vi "Multi Dut Cmd_Header Setting.vi"(8 "error in (no error)":errorcluster, 9 "Test Seq":i32(ring) items=["C1_C2_C3", "C2_C1_C3", "C3_C2_C1"], 11 "WS1050/51":bool=TRUE) -> (0 "error out":errorcluster, 1 "Cmd 3":string[](array[string]), 2 "Name 3":string[](array[string]), 3 "Name Header":string[](array[string]), 4 "Cmd 2":string[](array[string]), 5 "Name 2":string[](array[string]), 6 "Cmd 1":string[](array[string]), 7 "Name 1":string[](array[string]))   [LabVIEW 2012]
panel:
  in  "Cmd 51":string[](array[string])=["00", "01", "00", "02", "00", "04", "00", "08", "04", "0C", "08", "10", "0C", "14", "10", "18", "14", "1C", "18", "20", "1C", "24", "20", "28", "24", "2C", "28", "2F", "00"]
  in  "Name 51":string[](array[string])=["Min", "F1", "F1_OFF", "F2", "F2_OFF", "S1", "S1_OFF", "S2", "S2_OFF", "S3", "S3_OFF", "S4", "S4_OFF", "S5", "S5_OFF", "S6", "S6_OFF", "S7", "S7_OFF", "S8", "S8_OFF", "S9", "S9_OFF", "S10", "S10_OFF", "S11", "S11_OFF", "S11_F12", "Min2"]
  in  "Cmd 50":string[](array[string])=["00", "01", "00", "02", "00", "04", "00", "08", "04", "0C", "08", "10", "0C", "14", "10", "18", "14", "1C", "18", "20", "1C", "24", "20", "28", "24", "2C", "28", "30", "2C", "34", "30", "38", "34", "3B", "00"]
  in  "Name 50":string[](array[string])=["Min", "F1", "F1_OFF", "F2", "F2_OFF", "S1", "S1_OFF", "S2", "S2_OFF", "S3", "S3_OFF", "S4", "S4_OFF", "S5", "S5_OFF", "S6", "S6_OFF", "S7", "S7_OFF", "S8", "S8_OFF", "S9", "S9_OFF", "S10", "S10_OFF", "S11", "S11_OFF", "S12", "S12_OFF", "S13", "S13_OFF", "S14", "S14_OFF", "S14F12", "Min2"]
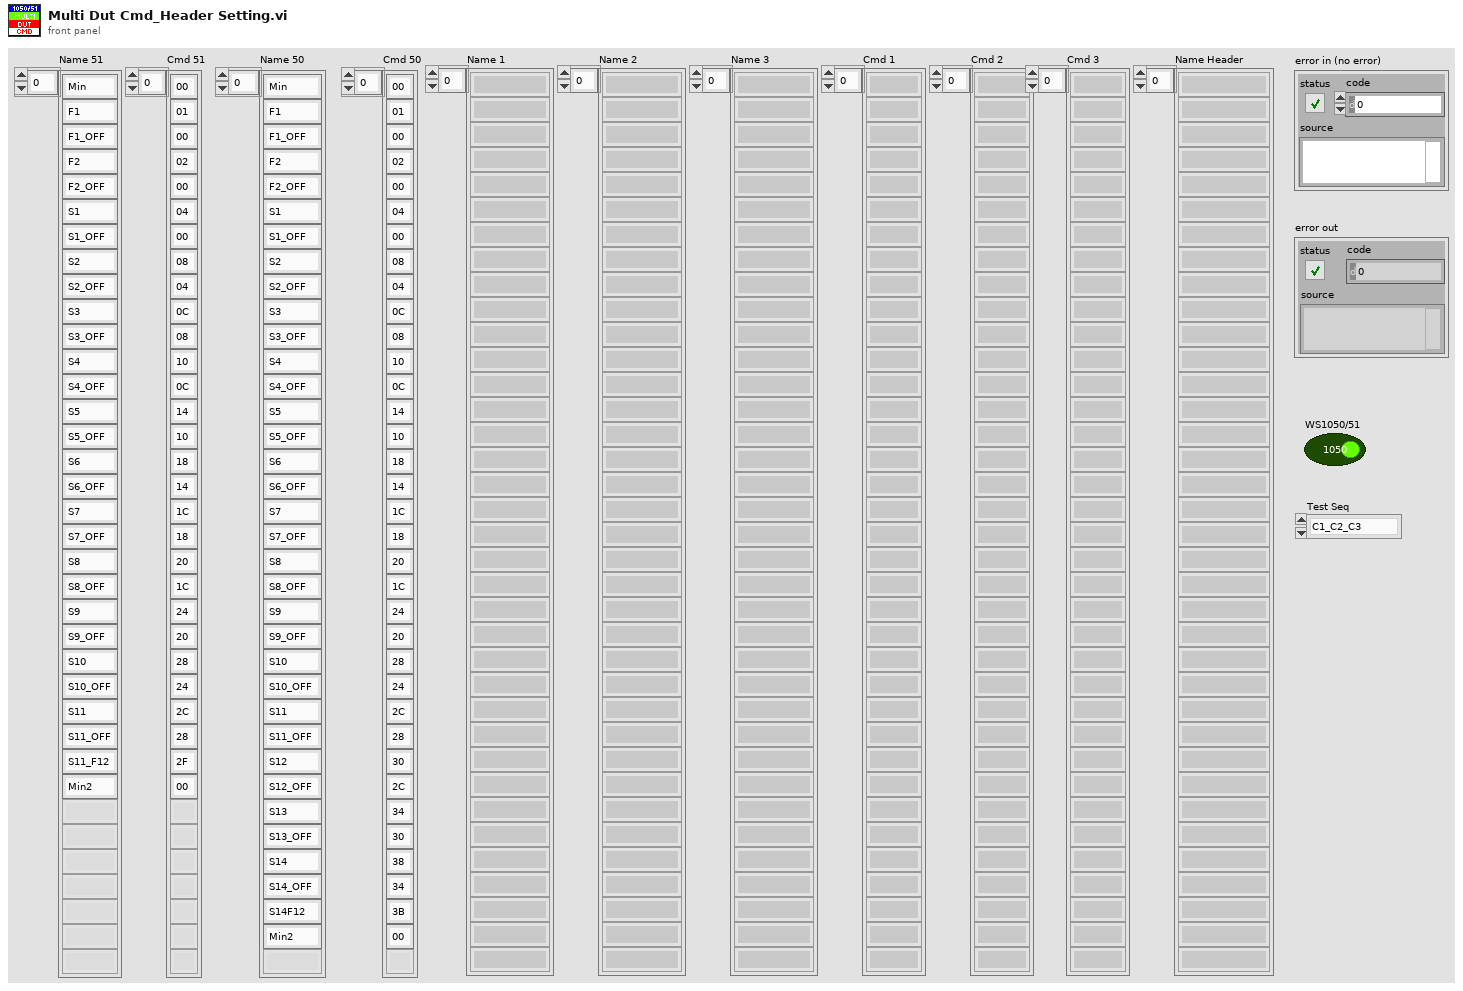
[diagram p1: front panel]
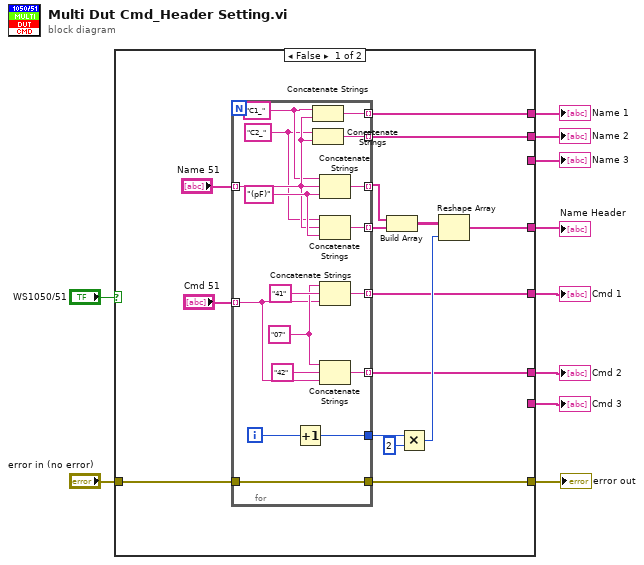
[diagram p0: block diagram]
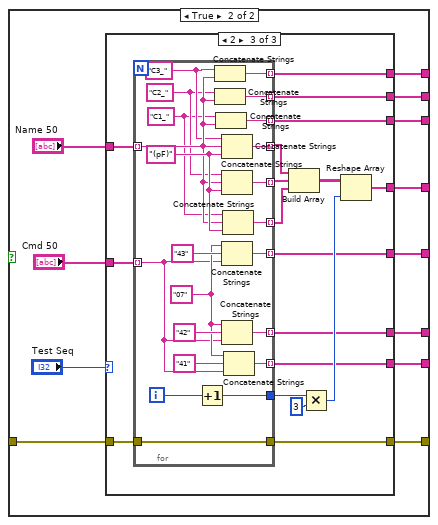
[diagram p2: hidden frame]
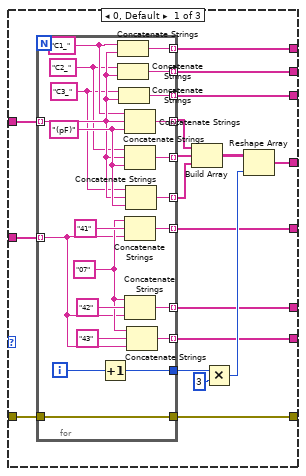
[diagram p3: hidden frame]
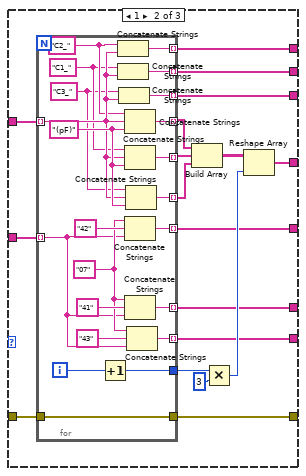
[diagram p4: hidden frame]
diagram:
  n1 = case shown="False" "WS1050/51" {
    tunnel: "error in (no error)" -> [w14 w52]
    tunnel: [w13 w51] -> w9
    tunnel: [w17 w50] -> w7
    tunnel: [w19 w49] -> w6
    tunnel: [w18 w48] -> w5
    tunnel: [_ w47] -> w4
    tunnel: [w12 w46] -> w3
    tunnel: [w11 w45] -> w2
    tunnel: [_ w44] -> w1
    frame False {
      n2 = for {
        tunnel: "Name 51" -> [w29] mode=indexing
        tunnel: [w42] -> w20 mode=indexing
        tunnel: [w41] -> w21 mode=indexing
        tunnel: "Cmd 51" -> [w35] mode=indexing
        tunnel: [w39] -> w12 mode=indexing
        tunnel: [w37] -> w11 mode=indexing
        tunnel: [w31] -> w19 mode=indexing
        tunnel: [w33] -> w24
        tunnel: [w30] -> w18 mode=indexing
        tunnel: w14 -> [w26]
        tunnel: [w26] -> w13
        i -> [w32]
        w27 = "C2_" ("string")
        w34 = "(pF)" ("string")
        w28 = "C1_" ("string")
        w36 = "07" ("string")
        n3 = Increment(x=w32) -> (x+1=w33:i32)
        n4 = Concatenate Strings(w28, w29) -> (w31:string)
        n5 = Concatenate Strings(w27, w29) -> (w30:string)
        n6 = Concatenate Strings(w28, w29, w34) -> (w42:string)
        n7 = Concatenate Strings(w27, w29, w34) -> (w41:string)
        n8 = Concatenate Strings(w36, "41" ("string"), w35) -> (w39:string)
        n9 = Concatenate Strings(w36, "42" ("string"), w35) -> (w37:string)
      }
      n10 = Build Array(w20, w21) -> (w22:string[][])
      n11 = Multiply(x=w24, y=2) -> (x*y=w23:i32)
      n12 = Reshape Array(w22, w23) -> (w17:string[])
    }
    frame True {
      n13 = case shown="2" "Test Seq" {
        tunnel: "Name 50" -> [w72 w112 w152]
        tunnel: "Cmd 50" -> [w71 w111 w151]
        tunnel: w52 -> [w63 w103 w143]
        tunnel: [w62 w102 w142] -> w51
        tunnel: [w61 w101 w141] -> w50
        tunnel: [w60 w100 w140] -> w49
        tunnel: [w59 w99 w139] -> w48
        tunnel: [w58 w98 w138] -> w47
        tunnel: [w57 w97 w137] -> w46
        tunnel: [w56 w96 w136] -> w45
        tunnel: [w55 w95 w135] -> w44
        frame 0, Default {
          n14 = for {
            tunnel: w72 -> [w78] mode=indexing
            tunnel: [w94] -> w70 mode=indexing
            tunnel: [w93] -> w69 mode=indexing
            tunnel: [w92] -> w68 mode=indexing
            tunnel: w71 -> [w85] mode=indexing
            tunnel: [w90] -> w57 mode=indexing
            tunnel: [w88] -> w56 mode=indexing
            tunnel: [w84] -> w55 mode=indexing
            tunnel: [w80] -> w60 mode=indexing
            tunnel: [w82] -> w65
            tunnel: [w79] -> w59 mode=indexing
            tunnel: [w77] -> w58 mode=indexing
            tunnel: w63 -> [w73]
            tunnel: [w73] -> w62
            i -> [w81]
            w74 = "C3_" ("string")
            w75 = "C2_" ("string")
            w83 = "(pF)" ("string")
            w76 = "C1_" ("string")
            w87 = "07" ("string")
            n15 = Increment(x=w81) -> (x+1=w82:i32)
            n16 = Concatenate Strings(w76, w78) -> (w80:string)
            n17 = Concatenate Strings(w75, w78) -> (w79:string)
            n18 = Concatenate Strings(w74, w78) -> (w77:string)
            n19 = Concatenate Strings(w76, w78, w83) -> (w94:string)
            n20 = Concatenate Strings(w75, w78, w83) -> (w93:string)
            n21 = Concatenate Strings(w87, "41" ("string"), w85) -> (w90:string)
            n22 = Concatenate Strings(w87, "42" ("string"), w85) -> (w88:string)
            n23 = Concatenate Strings(w74, w78, w83) -> (w92:string)
            n24 = Concatenate Strings(w87, "43" ("string"), w85) -> (w84:string)
          }
          n25 = Build Array(w70, w69, w68) -> (w67:string[][])
          n26 = Multiply(x=w65, y=3) -> (x*y=w66:i32)
          n27 = Reshape Array(w67, w66) -> (w61:string[])
        }
        frame 1 {
          n28 = for {
            tunnel: w112 -> [w118] mode=indexing
            tunnel: [w134] -> w110 mode=indexing
            tunnel: [w133] -> w109 mode=indexing
            tunnel: [w132] -> w108 mode=indexing
            tunnel: w111 -> [w125] mode=indexing
            tunnel: [w130] -> w97 mode=indexing
            tunnel: [w128] -> w96 mode=indexing
            tunnel: [w124] -> w95 mode=indexing
            tunnel: [w120] -> w100 mode=indexing
            tunnel: [w122] -> w105
            tunnel: [w119] -> w99 mode=indexing
            tunnel: [w117] -> w98 mode=indexing
            tunnel: w103 -> [w113]
            tunnel: [w113] -> w102
            i -> [w121]
            w114 = "C3_" ("string")
            w115 = "C1_" ("string")
            w123 = "(pF)" ("string")
            w116 = "C2_" ("string")
            w127 = "07" ("string")
            n29 = Increment(x=w121) -> (x+1=w122:i32)
            n30 = Concatenate Strings(w116, w118) -> (w120:string)
            n31 = Concatenate Strings(w115, w118) -> (w119:string)
            n32 = Concatenate Strings(w114, w118) -> (w117:string)
            n33 = Concatenate Strings(w116, w118, w123) -> (w134:string)
            n34 = Concatenate Strings(w115, w118, w123) -> (w133:string)
            n35 = Concatenate Strings(w127, "42" ("string"), w125) -> (w130:string)
            n36 = Concatenate Strings(w127, "41" ("string"), w125) -> (w128:string)
            n37 = Concatenate Strings(w114, w118, w123) -> (w132:string)
            n38 = Concatenate Strings(w127, "43" ("string"), w125) -> (w124:string)
          }
          n39 = Build Array(w110, w109, w108) -> (w107:string[][])
          n40 = Multiply(x=w105, y=3) -> (x*y=w106:i32)
          n41 = Reshape Array(w107, w106) -> (w101:string[])
        }
        frame 2 {
          n42 = for {
            tunnel: w152 -> [w158] mode=indexing
            tunnel: [w174] -> w150 mode=indexing
            tunnel: [w173] -> w149 mode=indexing
            tunnel: [w172] -> w148 mode=indexing
            tunnel: w151 -> [w165] mode=indexing
            tunnel: [w170] -> w137 mode=indexing
            tunnel: [w168] -> w136 mode=indexing
            tunnel: [w164] -> w135 mode=indexing
            tunnel: [w160] -> w140 mode=indexing
            tunnel: [w162] -> w145
            tunnel: [w159] -> w139 mode=indexing
            tunnel: [w157] -> w138 mode=indexing
            tunnel: w143 -> [w153]
            tunnel: [w153] -> w142
            i -> [w161]
            w154 = "C1_" ("string")
            w155 = "C2_" ("string")
            w163 = "(pF)" ("string")
            w156 = "C3_" ("string")
            w167 = "07" ("string")
            n43 = Increment(x=w161) -> (x+1=w162:i32)
            n44 = Concatenate Strings(w156, w158) -> (w160:string)
            n45 = Concatenate Strings(w155, w158) -> (w159:string)
            n46 = Concatenate Strings(w154, w158) -> (w157:string)
            n47 = Concatenate Strings(w156, w158, w163) -> (w174:string)
            n48 = Concatenate Strings(w155, w158, w163) -> (w173:string)
            n49 = Concatenate Strings(w167, "43" ("string"), w165) -> (w170:string)
            n50 = Concatenate Strings(w167, "42" ("string"), w165) -> (w168:string)
            n51 = Concatenate Strings(w154, w158, w163) -> (w172:string)
            n52 = Concatenate Strings(w167, "41" ("string"), w165) -> (w164:string)
          }
          n53 = Build Array(w150, w149, w148) -> (w147:string[][])
          n54 = Multiply(x=w145, y=3) -> (x*y=w146:i32)
          n55 = Reshape Array(w147, w146) -> (w141:string[])
        }
      }
    }
  }
  "error out" <- w9
  "Name Header" <- w7
  "Name 1" <- w6
  "Name 2" <- w5
  "Name 3" <- w4
  "Cmd 1" <- w3
  "Cmd 2" <- w2
  "Cmd 3" <- w1
